vi "SaveControlsToSettingsFile.vi"(5 "Prefix":string="Name", 7 "VI Refnum":refnum<vi>, 9 "Save?":bool, 10 "ControlRefArray":refnum<vi>[](array[refnum]), 11 "Save Path":path) -> (3 "Saved Settings Path":path)   [LabVIEW 2015]
uses:
  <vilib>/Utility/file.llb/Write Delimited Spreadsheet (string).vi
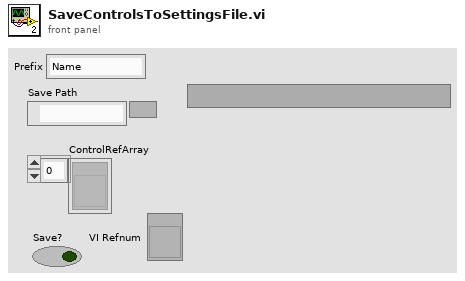
[diagram p1: front panel]
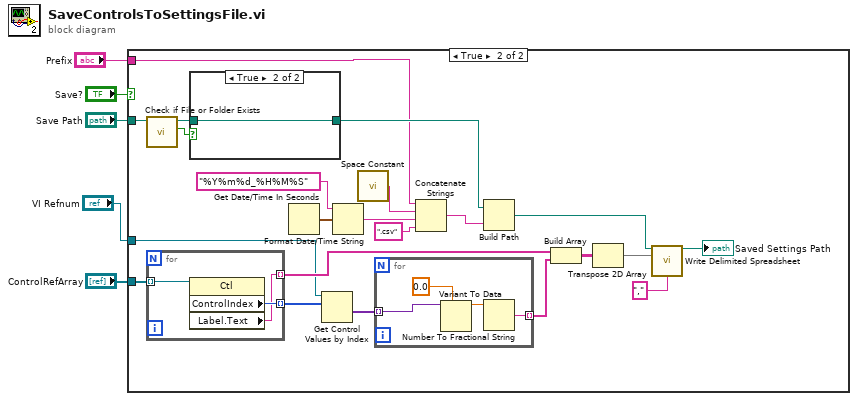
[diagram p0: block diagram]
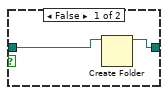
[diagram p3: hidden frame]
diagram:
  n1 = case shown="True" "Save?" {
    tunnel: "ControlRefArray" -> [_ w27]
    tunnel: "Save Path" -> [_ w13]
    tunnel: "VI Refnum" -> [_ w8]
    tunnel: "Prefix" -> [_ w7]
    frame False {
    }
    frame True {
      n2 = call <vilib>:"Check if File or Folder Exists.vi"("path"=w13) -> ("file or folder exists?"=w21:bool, "dup path"=w20:path)  [unwired: 8 in, 1 out]
      n3 = for {
        tunnel: w27 -> [w34] mode=indexing
        tunnel: [w33] -> w26 mode=indexing
        tunnel: [w32] -> w25 mode=indexing
        n4 = property class="Ctl"(reference=w34) -> ("ControlIndex"=w33:i32, "Label.Text"=w32:string)  [unwired: 1 in, 2 out]
      }
      n5 = case shown="True" w21 {
        tunnel: w20 -> [w36 w37]
        tunnel: [w35 w37] -> w17
        frame False {
          n6 = Create Folder(path (use dialog)=w36) -> (created path=w35:path)  [unwired: 2 in, 2 out]
        }
        frame True {
        }
      }
      n7 = Get Date/Time In Seconds() -> (seconds since 1Jan1904=w19:timestamp)
      n8 = Get Control Values by Index(0:w8, 1:w26) -> (10:w24:variant[])  [unwired: 1 in, 1 out]
      n9 = Format Date/Time String(time format string (%c)="%Y%m%d_%H%M%S", seconds (now)=w19) -> (date/time string=w16:string)  [unwired: 1 in]
      n10 = call <vilib>:"Space Constant.vi"() -> ("String"=w6:string)
      n11 = for {
        tunnel: w24 -> [w31] mode=indexing
        tunnel: [w28] -> w23 mode=indexing
        n12 = Variant To Data(type=0.0, Variant=w31) -> (data=w29:dbl)  [unwired: 1 in, 1 out]
        n13 = Number To Fractional String(number=w29) -> (F-format string=w28:string)  [unwired: 3 in]
      }
      n14 = Concatenate Strings(w7, w6, w16, ".csv" ("string")) -> (w14:string)
      n15 = Build Path(base path=w17, name or relative path=w14) -> (appended path=w12:path)
      n16 = Build Array(w25, w23) -> (w22:string[][])
      n17 = Transpose 2D Array(2D array=w22) -> (transposed array=w11:string[][])
      n18 = call-poly <vilib>:"Write Delimited Spreadsheet.vi"("file path (dialog if empty)"=w12, "2D data"=w11, "delimiter (\\t)"="," ("delimiter (\\t)")) -> ("new file path (Not A Path if cancelled)"=→"Saved Settings Path":path)  [unwired: 11 in, 1 out]
    }
  }
